vi "bigcryo_H-zero.vi"(9 "Rate [T/min]":dbl=0.5, 11 "Magnet Power supply":refnum<visa-resource-name>) -> ()   [LabVIEW 2019]
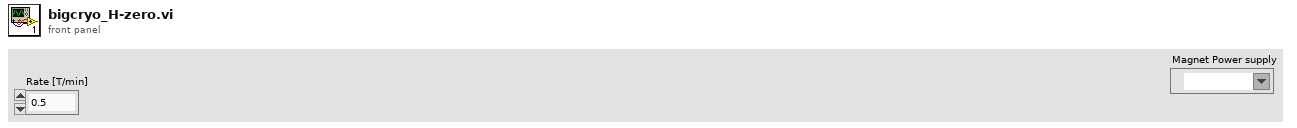
[diagram p1: front panel]
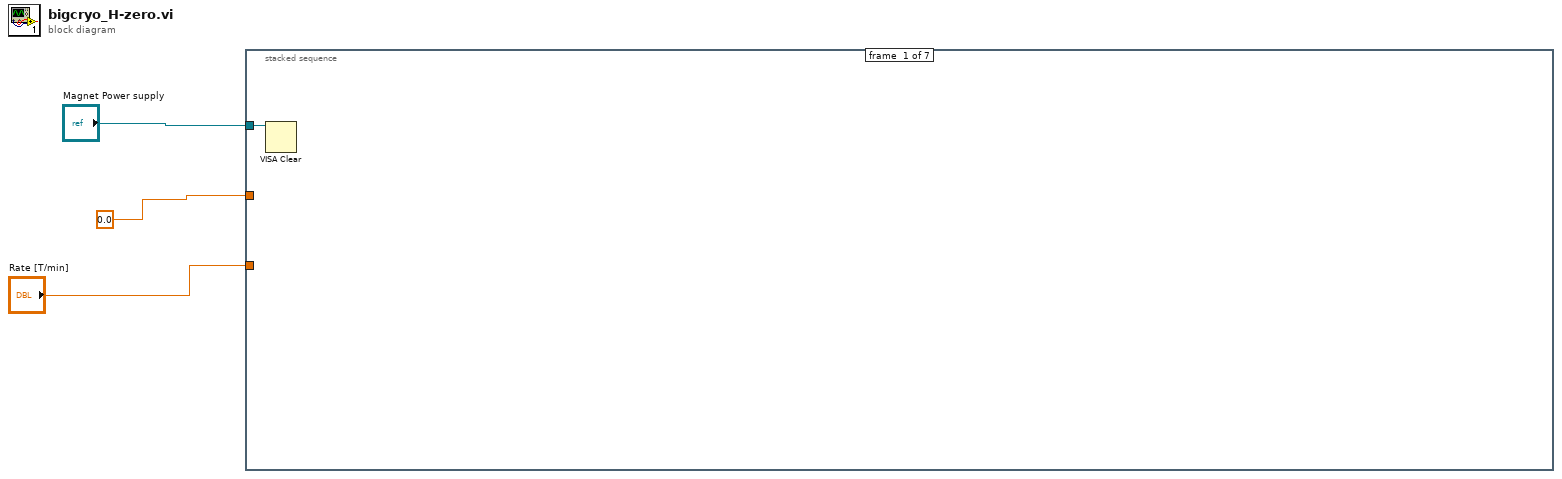
[diagram p0: block diagram]
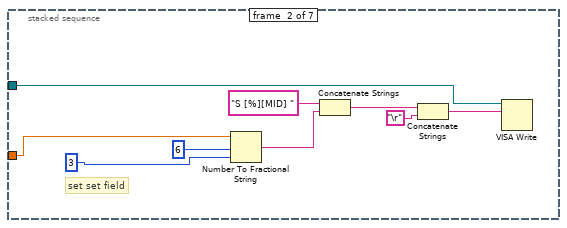
[diagram p2: hidden frame]
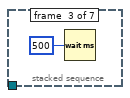
[diagram p3: hidden frame]
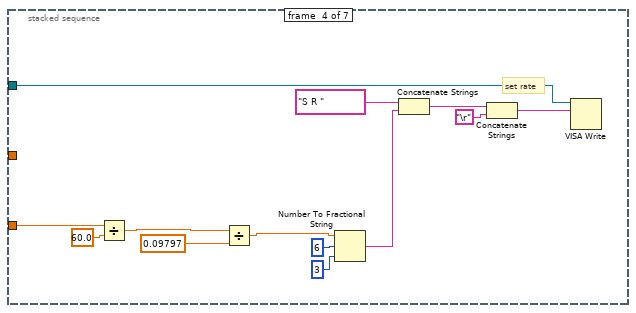
[diagram p4: hidden frame]
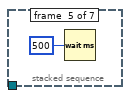
[diagram p5: hidden frame]
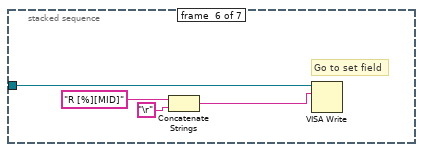
[diagram p6: hidden frame]
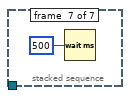
[diagram p7: hidden frame]
diagram:
  n1 = stacked-sequence {
    tunnel: "Magnet Power supply" -> [w4 w7 _ w25 _ w30 _]
    tunnel: "Rate [T/min]" -> [_ _ _ w15 _ _ _]
    tunnel: 0.0 ("Set Field [T]") -> [_ w5 _ _ _ _ _]
    frame #0 {
      n2 = VISA Clear(VISA resource name=w4) -> ()  [unwired: 1 in, 2 out]
    }
    frame #1 {
      # "set set field"
      n3 = Number To Fractional String(number=w5, width (-)=i16 6, precision (6)=i16 3) -> (F-format string=w10:string)  [unwired: 1 in]
      n4 = Concatenate Strings("S [%][MID] " ("string"), w10) -> (w6:string)
      n5 = Concatenate Strings(w6, "\r") -> (w9:string)
      n6 = VISA Write(VISA resource name=w7, write buffer=w9) -> ()  [unwired: 1 in, 3 out]
    }
    frame #2 {
      n7 = Wait (ms)(milliseconds to wait=500) -> ()  [unwired: 1 out]
    }
    frame #3 {
      # "set rate"
      n8 = Divide(x=w15, y=60.0) -> (x/y=w20:dbl)
      n9 = Divide(x=w20, y=0.09797) -> (x/y=w18:dbl)
      n10 = Number To Fractional String(number=w18, width (-)=i16 6, precision (6)=i16 3) -> (F-format string=w23:string)  [unwired: 1 in]
      n11 = Concatenate Strings("S R " ("string"), w23) -> (w22:string)
      n12 = Concatenate Strings(w22, "\r") -> (w27:string)
      n13 = VISA Write(VISA resource name=w25, write buffer=w27) -> ()  [unwired: 1 in, 3 out]
    }
    frame #4 {
      n14 = Wait (ms)(milliseconds to wait=500) -> ()  [unwired: 1 out]
    }
    frame #5 {
      # "Go to set field"
      n15 = Concatenate Strings("R [%][MID]" ("data"), "\r") -> (w32:string)
      n16 = VISA Write(VISA resource name=w30, write buffer=w32) -> ()  [unwired: 1 in, 3 out]
    }
    frame #6 {
      n17 = Wait (ms)(milliseconds to wait=500) -> ()  [unwired: 1 out]
    }
  }
